vi "LJM_eStreamStart.vi"(0 "Handle In":i32, 1 "aScanList":i32[](array[numeric]), 5 "ScansPerRead":i32, 7 "NumAddresses (-1 = Auto-Detect)":i32=-1, 9 "ScanRate":dbl format="%_2f", 11 "error in":errorcluster) -> (4 "Handle Out":i32, 6 "ScansPerRead Out":i32, 8 "NumReadAddresses":i32, 10 "Actual ScanRate":dbl format="%.3f", 14 "Actual SampleRate":dbl format="%.3f", 15 "error out":errorcluster)   [LabVIEW 2020]
uses:
  Library/Frameworks/LabJackM.framework
panel:
  # "This is the number of addresses that\nwill return stream data.\nStream_Out# channels are included in\nscan list, but do not return any data."
  # "1/22/2015:  Default value of NumAddresses changed to -1 which\nequates to Auto-Detect.  If NumAddresses = -1, then the NumAddresses\ncontrol is ignored and the size of aScanList is used to determine how many\naddresses there are.  Also added ScansPerRead & NumAddresses outputs that\ncan be wired to eStreamRead.  Also moved the terminal location of\nActual ScanRate."
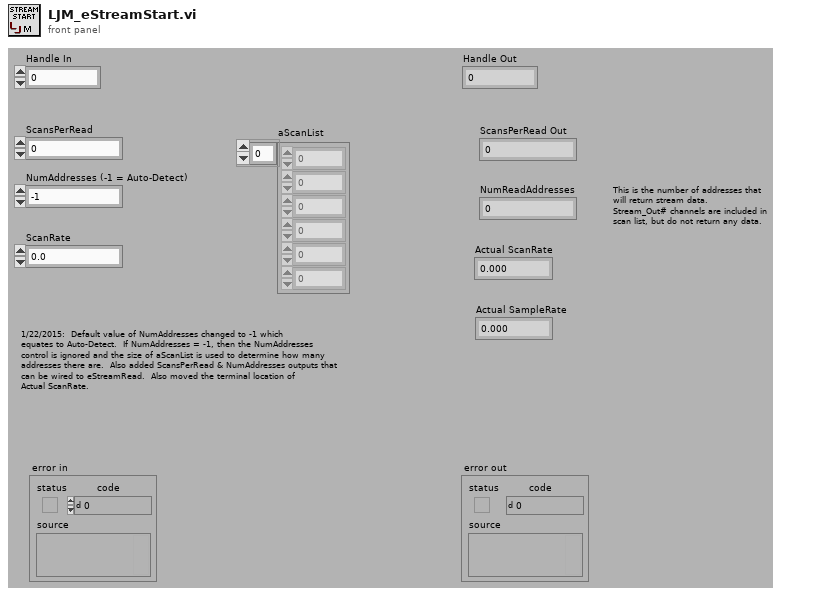
[diagram p1: front panel]
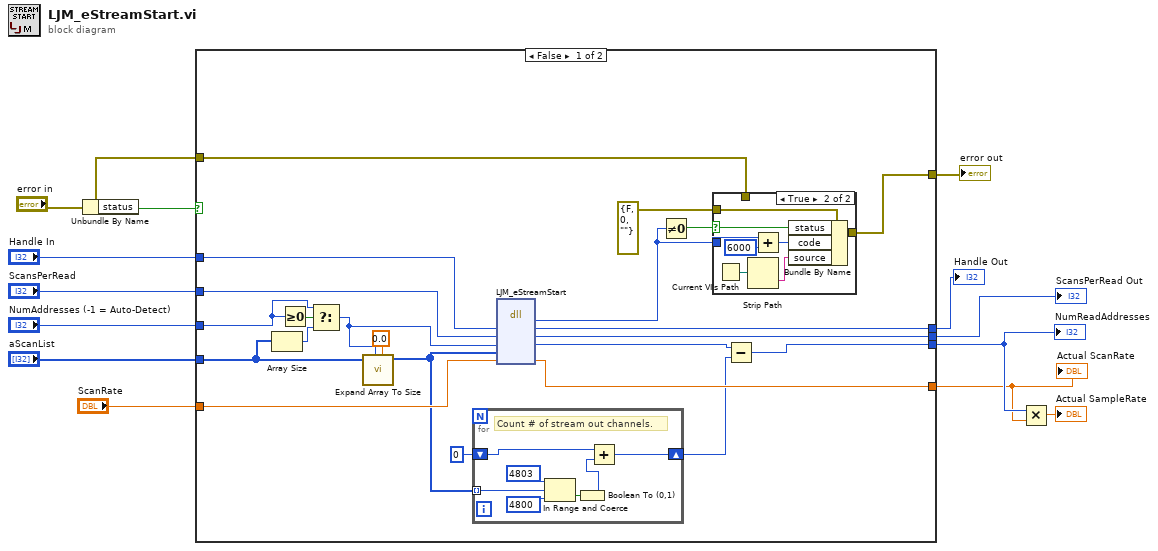
[diagram p0: block diagram]
diagram:
  n1 = Unbundle By Name("error in") -> ("status"=w13:bool)
  n2 = case shown="False" w13 {
    tunnel: "error in" -> [w31 w56]
    tunnel: [w32 w56] -> w12
    tunnel: [w30 w55] -> w11
    tunnel: "Handle In" -> [w29 w55]
    tunnel: "ScansPerRead" -> [w28 w52]
    tunnel: "NumAddresses (-1 = Auto-Detect)" -> [w22 w53]
    tunnel: "aScanList" -> [w20 _]
    tunnel: "ScanRate" -> [w26 w54]
    tunnel: [w25 w54] -> w2
    tunnel: [w14 w53] -> w3
    tunnel: [w19 w52] -> w1
    frame False {
      n3 = Array Size(array=w20) -> (size(s)=w23:i32)
      n4 = Greater Or Equal To 0?(x=w22) -> (x >= 0?=w24:bool)
      n5 = Select(t=w22, s=w24, f=w23) -> (s? t:f=w21:i32)
      n6 = call "Expand Array To Size.vi"("Default Value"=0.0, "# Elements"=w21, "I32 Array In"=w20) -> ("I32 Array Out"=w18:i32[])  [unwired: 4 in, 4 out]
      n7 = for {
        tunnel: w18 -> [w42] mode=indexing
        shift-right: [w38] -> w15
        shift-left: i16 0 -> [w36]
        # "Count # of stream out channels."
        n8 = In Range and Coerce(upper limit=4803, x=w42, lower limit=4800) -> (In Range?=w39:bool)  [unwired: 1 out]
        n9 = Boolean To (0,1)(Boolean=w39) -> (0, 1=w37:i16)
        n10 = Add(x=w36, y=w37) -> (x+y=w38:i16)
      }
      n11 = dll-call lib="Library/Frameworks/LabJackM.framework" fn="LJM_eStreamStart"("Handle"=w29, "ScansPerRead"=w28, "NumAddresses"=w21, "aScanList"=w18, "ScanRate"=w26) -> ("return type"=w35:i32, "Handle"=w30:i32, "ScansPerRead"=w19:i32, "NumAddresses"=w16:i32, "ScanRate"=w25:dbl)  [unwired: 4 in, 2 out]
      n12 = Not Equal To 0?(x=w35) -> (x != 0?=w34:bool)
      n13 = case shown="True" w34 {
        selector: w34 -> [_ w50]
        tunnel: [w43 w51] -> w32
        tunnel: errorcluster {"status"=FALSE, "code"=0, "source"=""} ("error IO") -> [_ w49]
        tunnel: w35 -> [_ w45]
        tunnel: w31 -> [w43 _]
        frame False {
        }
        frame True {
          n14 = Current VI's Path() -> (path=w47:path)
          n15 = Strip Path(path=w47) -> (name=w48:string)  [unwired: 1 out]
          n16 = Add(x=w45, y=6000) -> (x+y=w46:i32)
          n17 = Bundle By Name(cluster=w49, "status"=w50, "code"=w46, "source"=w48) -> (w51:errorcluster)
        }
      }
      n18 = Subtract(x=w16, y=w15) -> (x-y=w14:i32)
    }
    frame True {
    }
  }
  "error out" <- w12
  "Handle Out" <- w11
  "Actual ScanRate" <- w2
  "NumReadAddresses" <- w3
  "ScansPerRead Out" <- w1
  n19 = Multiply(x=w3, y=w2) -> (x*y=→"Actual SampleRate":dbl)
